vi "ReadFlag.vi"(8 "error in (no error)":errorcluster, 11 "Room Number":i32) -> (0 "error out":errorcluster, 2 "Flags JSON":string)   [LabVIEW 2015, in "RestApi.lvlib"]
uses:
  RestApi.lvlib
  FGVAction.ctl
  <vilib>/httpClient/LabVIEWHTTPClient.lvlib
panel:
  out "URL":string
  out "headers":string
  # "http://127.0.0.1:8001/WebService1/ReadFlag?Room={value}"
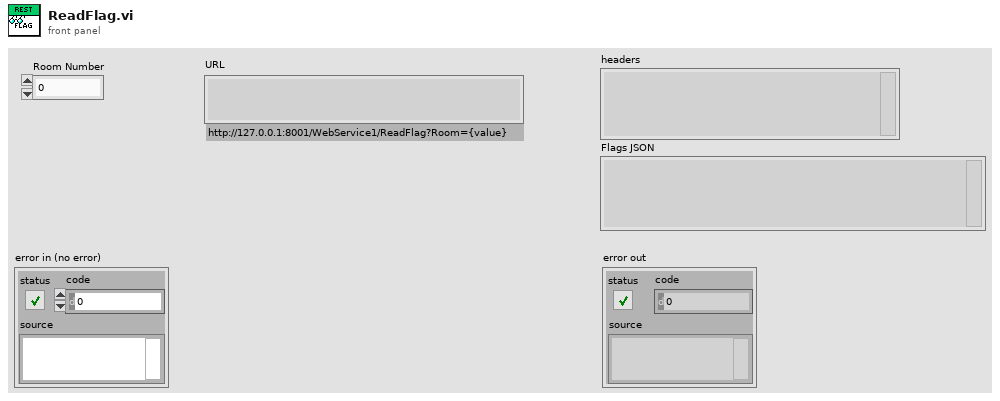
[diagram p1: front panel]
types:
  T1 = typedef "FGVAction.ctl" = enum16{"Get", "Set"}
  T2 = typedef "LabVIEWHTTPClient.lvlib/ClientHandle.ctl" = refnum<k1>
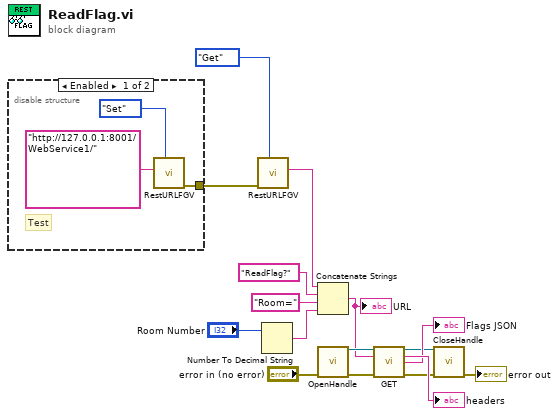
[diagram p0: block diagram]
diagram:
  n1 = disable-structure shown="Enabled" {
    disable-tunnel: [w17 _] -> w9
    frame Enabled {
      # "Test"
      n2 = call "RestURLFGV.vi"("Action"=FGVAction."Set", "URL"="http://127.0.0.1:8001/WebService1/" ("url")) -> ("error out"=w17:errorcluster)  [unwired: 8 in, 1 out]
    }
    frame Disabled {
    }
  }
  n3 = call "RestURLFGV.vi"("Action"=FGVAction."Get", "error in (no error)"=w9) -> ("URL"=w2:string)  [unwired: 8 in, 1 out]
  n4 = Number To Decimal String(number="Room Number") -> (decimal integer string=w6:string)  [unwired: 1 in]
  n5 = Concatenate Strings(w2, "ReadFlag?" ("string"), "Room=" ("string"), w6) -> (w3:string)
  "URL" <- w3
  n6 = call <vilib>:"OpenHandle.vi"("error in (no error)"="error in (no error)") -> ("client handle out"=w16:T2, "error out"=w11:errorcluster)  [unwired: 13 in]
  n7 = call <vilib>:"GET.vi"("client handle"=w16, "url"=w3, "error in (no error)"=w11) -> ("client handle out"=w13:T2, "headers"=→"headers":string, "body"=→"Flags JSON":string, "error out"=w12:errorcluster)  [unwired: 9 in]
  n8 = call <vilib>:"CloseHandle.vi"("client handle"=w13, "error in (no error)"=w12) -> ("error out"=→"error out":errorcluster)  [unwired: 13 in]
